vi "pathplan_vertices_send - 副本.vi"(1 "vertices":dbl[][](array[numeric])=[[5650.0, 5700.0, 5675.0, 5651.0, 5626.0, 5602.0, 5577.0, 5553.0, 5529.0, 5504.0], [1700.0, 1750.0, 1793.0, 1837.0, 1880.0, 1924.0, 1968.0, 2011.0, 2055.0, 2099.0]], 2 "distance_all":dbl, 3 "angle_all":dbl[](array[numeric])=[45.0, 119.0, 119.0, 119.0, 119.0, 119.0, 119.0, 119.0, 119.0, 0.0], 4 "speed_max":dbl, 5 "写入串口":refnum<visa-resource-name>) -> (20 "路径规划数据写入缓冲区":string)   [LabVIEW 2016]
uses:
  <vilib>/imath/engines/lvmath2/RunTimeEngine/NodeEndStatement/NIMS_NodeEndStatement_Output.vi
  <instcachedir>/0/NIMS_NodeEndStatement_Output_53EC0D466D134D7ABD903AC30B43404B.lvgen/NIMS_NodeEndStatement_Output_53EC0D466D134D7ABD903AC30B43404B_015.vi
  <instcachedir>/0/NIMS_NodeEndStatement_Output_53EC0D466D134D7ABD903AC30B43404B.lvgen/NIMS_NodeEndStatement_Output_53EC0D466D134D7ABD903AC30B43404B_011.vi
  <vilib>/imath/engines/lvmath2/RunTimeEngine/ErrorHandling/NIMS_Finalize Error.vi
  <vilib>/imath/engines/lvmath2/RunTimeEngine/IndexRead/NIMS M($,S).vi
  <instcachedir>/0/NIMS M($,S)_3E5749BBB62E49528D4765A77F1F6D98.lvgen/NIMS M($,S)_3E5749BBB62E49528D4765A77F1F6D98_000.vi
  <vilib>/imath/engines/lvmath2/RunTimeEngine/ArithmeticOperatorToken/NIMS_ArithmeticOperator_minus.vi
  <instcachedir>/0/NIMS_ArithmeticOperator_minus_E3B65B1D26A44BB184AFDC5B3F458E3D.lvgen/NIMS_ArithmeticOperator_minus_E3B65B1D26A44BB184AFDC5B3F458E3D_003.vi
  <vilib>/imath/engines/lvmath2/RunTimeEngine/ErrorHandling/NIMS_Create Error From Enums.vi
  <vilib>/imath/engines/lvmath2/RunTimeEngine/IndexRead/NIMS V(S).vi
  <instcachedir>/0/NIMS V(S)_0488751826AF41519A22953C041130DC.lvgen/NIMS V(S)_0488751826AF41519A22953C041130DC_000.vi
  <vilib>/imath/engines/lvmath2/RunTimeEngine/BuiltInFunctions/abs/NIMS_abs(signed).vi
  <instcachedir>/0/NIMS_abs(signed)_C4FCB8E6058B49B797C7C8D53CA5F6EC.lvgen/NIMS_abs(signed)_C4FCB8E6058B49B797C7C8D53CA5F6EC_000.vi
  <vilib>/imath/engines/lvmath2/RunTimeEngine/BuiltInFunctions/length/NIMS_length(GM).vi
  <instcachedir>/0/NIMS_length(GM)_47CEC356FCE0482D9BA47DC61C99F2C7.lvgen/NIMS_length(GM)_47CEC356FCE0482D9BA47DC61C99F2C7_000.vi
  <vilib>/imath/engines/lvmath2/RunTimeEngine/IndexRead/NIMS M($,R2).vi
  <instcachedir>/0/NIMS M($,R2)_D9380E19261A4ADFB2D364AF6959C6EF.lvgen/NIMS M($,R2)_D9380E19261A4ADFB2D364AF6959C6EF_001.vi
  <vilib>/imath/engines/lvmath2/RunTimeEngine/RowToken/NIMS_RowToken_M_CV.vi
  <instcachedir>/0/NIMS_RowToken_M_CV_FA79F1D1D17D44459F3ED8E09EE8B625.lvgen/NIMS_RowToken_M_CV_FA79F1D1D17D44459F3ED8E09EE8B625_000.vi
  <vilib>/imath/engines/lvmath2/RunTimeEngine/BuiltInFunctions/size/NIMS_I32=size(GM,I32).vi
  <instcachedir>/0/NIMS_I32=size(GM,I32)_122058B1B3294FAEA5DC209B92B394E4.lvgen/NIMS_I32=size(GM,I32)_122058B1B3294FAEA5DC209B92B394E4_004.vi
  <vilib>/imathl/engines/lvmath/Functions/Error Handling/Create Error.vi
  <vilib>/imath/engines/lvmath2/RunTimeEngine/RangeToken/NIMS_Range_R2 - Integer.vi
  <instcachedir>/0/NIMS_Range_R2 - Integer_89B873E74E6E489885E44F751DD9C6BF.lvgen/NIMS_Range_R2 - Integer_89B873E74E6E489885E44F751DD9C6BF_000.vi
  <vilib>/imath/engines/lvmath2/RunTimeEngine/CommandStatement/MC_CommandStatement_break.vi
  <vilib>/imath/engines/lvmath2/RunTimeEngine/BuiltInFunctions/norm/NIMS_norm(GV,DBL).vi
  <instcachedir>/0/NIMS_norm(GV,DBL)_1268AFF3C646412B8C6EA3CE75D09042.lvgen/NIMS_norm(GV,DBL)_1268AFF3C646412B8C6EA3CE75D09042_000.vi
  <instcachedir>/0/NIMS_NodeEndStatement_Output_53EC0D466D134D7ABD903AC30B43404B.lvgen/NIMS_NodeEndStatement_Output_53EC0D466D134D7ABD903AC30B43404B_010.vi
  <instcachedir>/0/NIMS_NodeEndStatement_Output_53EC0D466D134D7ABD903AC30B43404B.lvgen/NIMS_NodeEndStatement_Output_53EC0D466D134D7ABD903AC30B43404B_005.vi
  <vilib>/imath/engines/lvmath2/RunTimeEngine/BuiltInFunctions/dot/NIMS_dot(GV,GV).vi
  <instcachedir>/0/NIMS_dot(GV,GV)_B9FAA411F4494E9B94D442721014A3FA.lvgen/NIMS_dot(GV,GV)_B9FAA411F4494E9B94D442721014A3FA_000.vi
  <instcachedir>/0/NIMS_NodeEndStatement_Output_53EC0D466D134D7ABD903AC30B43404B.lvgen/NIMS_NodeEndStatement_Output_53EC0D466D134D7ABD903AC30B43404B_009.vi
panel:
  in  "y":dbl
  in  "x":dbl
  in  "angle_z":sgl
  out "angle_send":dbl[](array[numeric])
  out "vertices_send":dbl[](array[numeric])
  out "speed_send":dbl[](array[numeric])
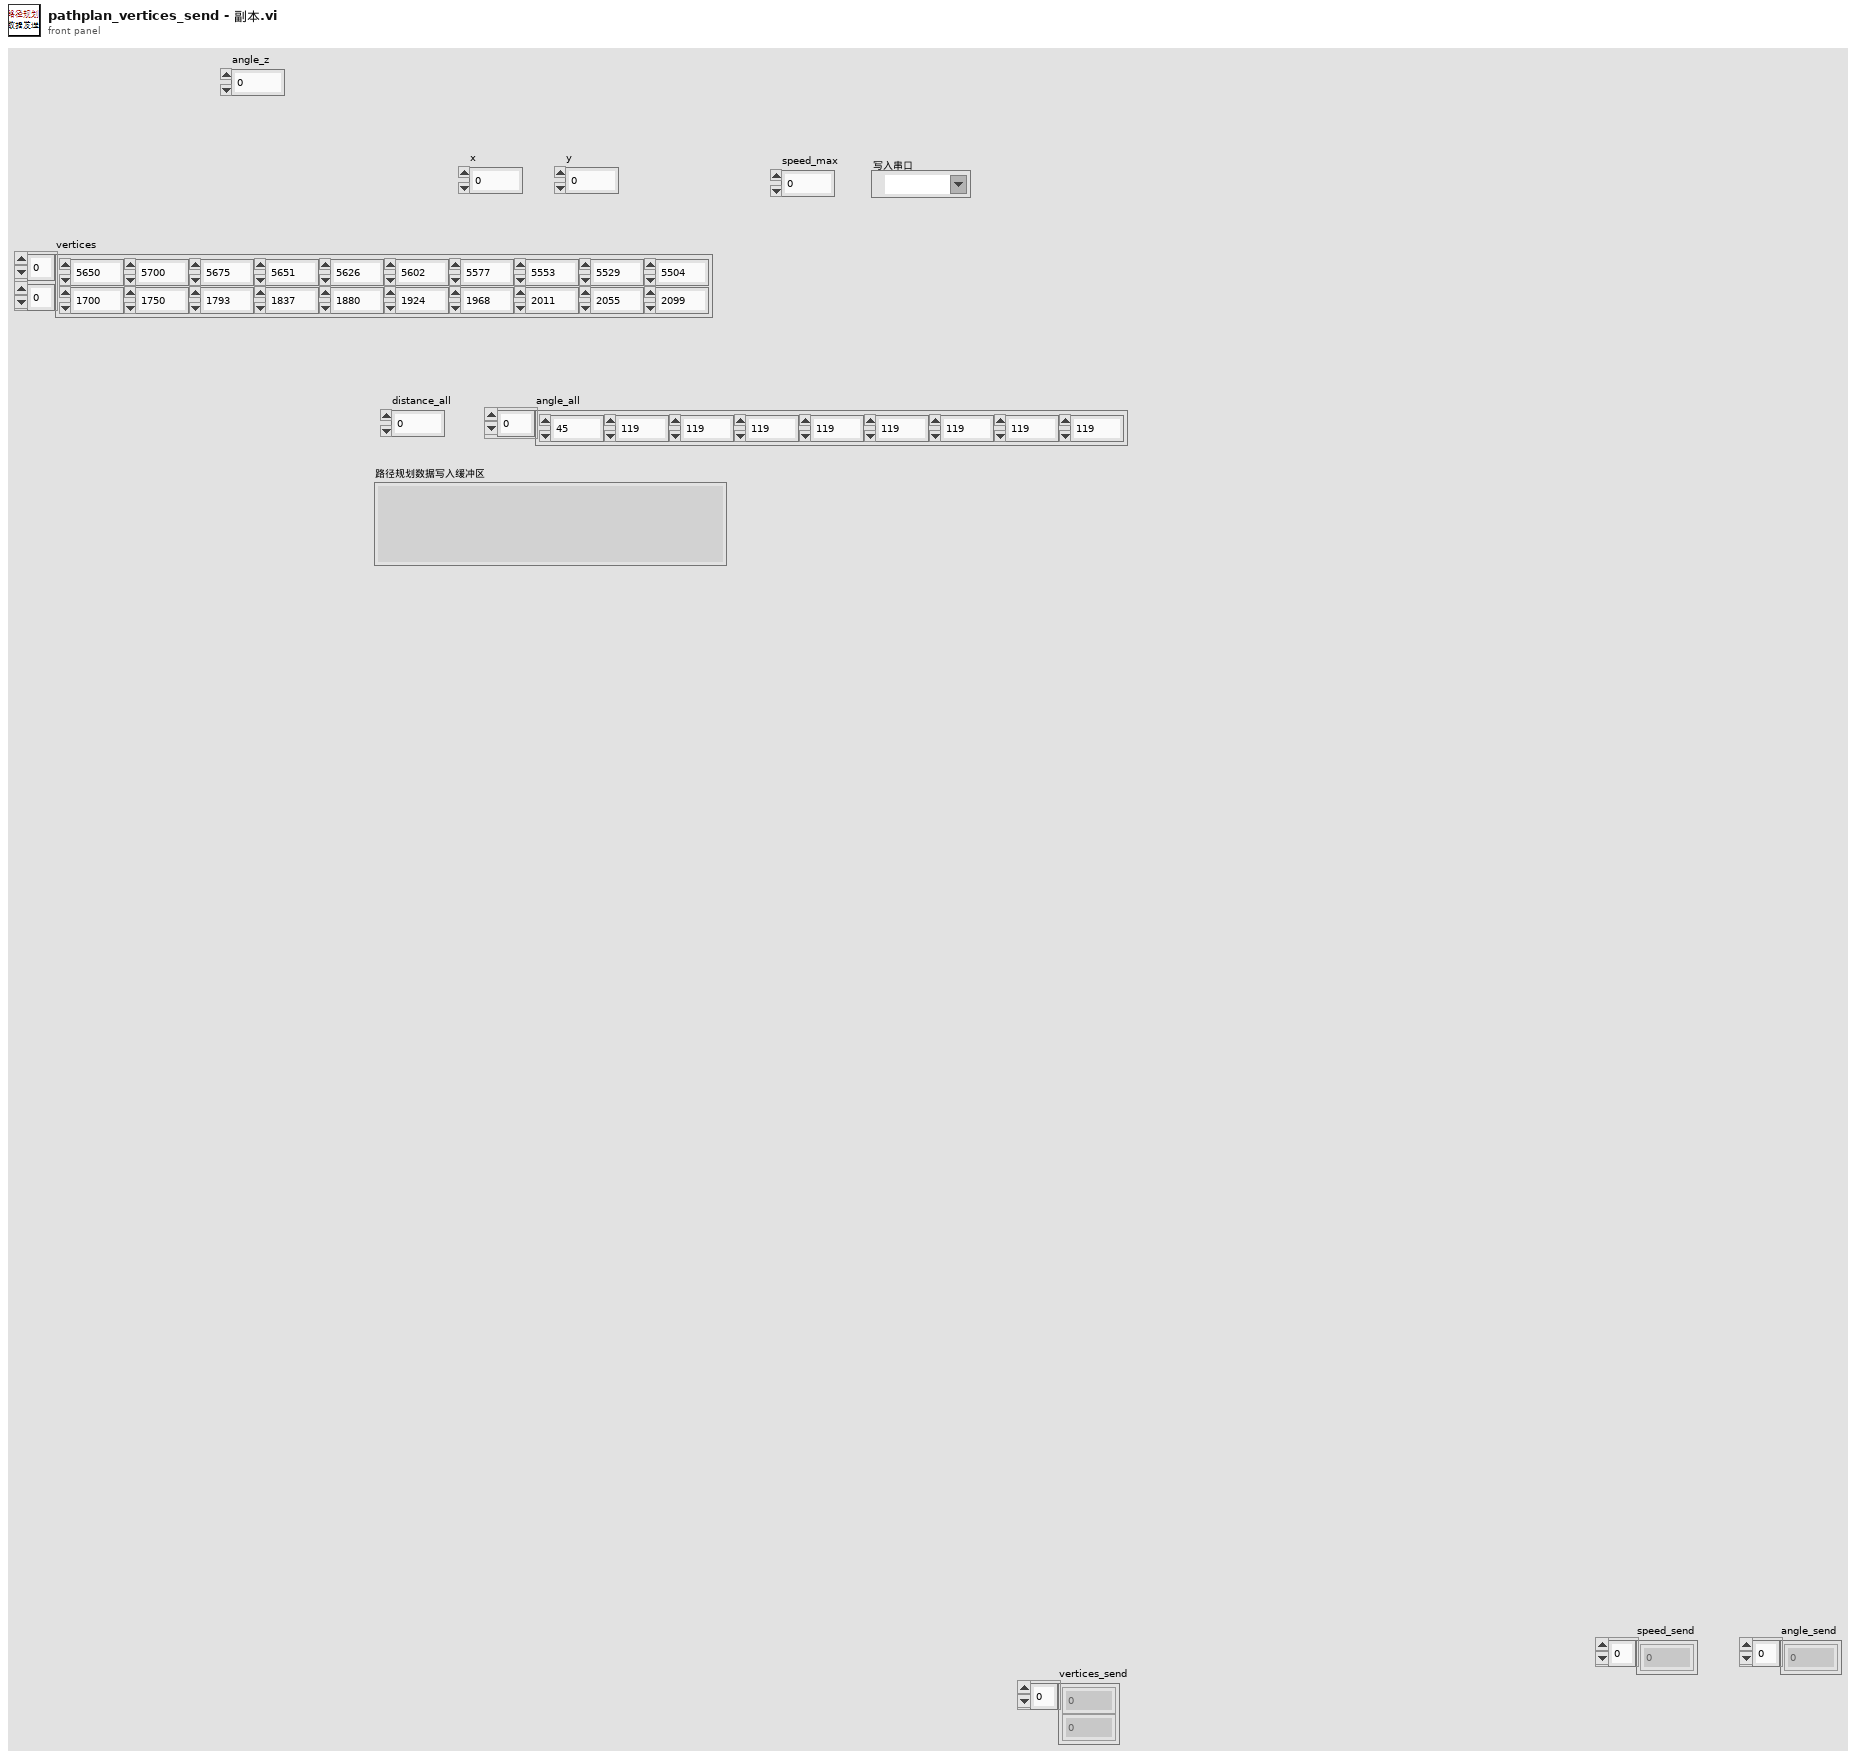
[diagram p1: front panel]
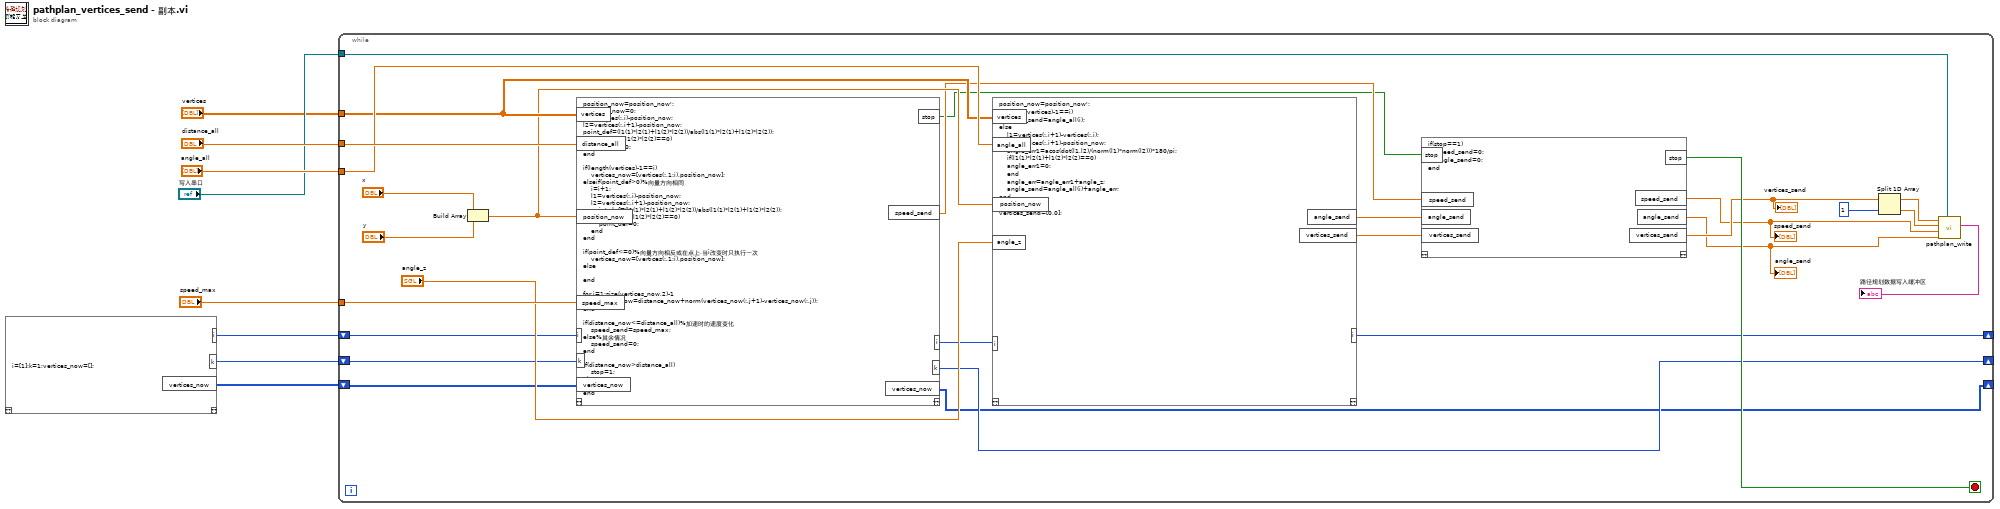
[diagram p0: block diagram]
diagram:
  n1 = mathscript code="i=[1];k=1;vertices_now=[];"() -> ("i"=w3:i32, "k"=w2:i32, "vertices_now"=w1:i32[][])  [unwired: 1 in, 1 out]
  n2 = while {
    tunnel: "vertices" -> [w34]
    tunnel: "distance_all" -> [w36]
    tunnel: "angle_all" -> [w35]
    shift-right: [w11] -> _
    shift-left: w3 -> [w13]
    tunnel: "speed_max" -> [w32]
    shift-right: [w14] -> _
    shift-left: w2 -> [w15]
    shift-right: [w9] -> _
    shift-left: w1 -> [w10]
    tunnel: "写入串口" -> [w20]
    stop <- w24 stop-if-true
    n3 = Build Array("x", "y") -> (w33:dbl[])
    n4 = mathscript code="position_now=position_now';\ndistance_now=0;\nl1=vertices(:,i)-position_now;\nl2=vertices(:,i+1)-position_now;\npoint_def=(l1(1)*l2(1)+l1(2)*l2(2))/abs(l1(1)*l2(1)+l1(2)*l2(2));\nif(l1(1)*l2(1)+l1(2)*l2(2)==0)\n    point_def=0;\nend\n\nif(length(vertices)-1==i)\n    vertices_now=[vertices(:,1:i),position_now];\nelseif(point_def>0)%向量方向相同\n    i=i+1;\n    l1=vertices(:,i)-position_now;\n    l2=vertices(:,i+1)-position_now;\n    point_def=(l1(1)*l2(1)+l1(2)*l2(2))/abs(l1(1)*l2(1)+l1(2)*l2(2));\n    if(l1(1)*l2(1)+l1(2)*l2(2)==0)\n        point_def=0;\n    end\nend\n\nif(point_def<=0)%向量方向相反或在点上,当i改变时只执行一次\n    vertices_now=[vertices(:,1:i),position_now];\nelse\n\nend\n\nfor j=1:size(vertices_now,2)-1\n    distance_now=distance_now+norm(vertices_now(:,j+1)-vertices_now(:,j));\nend\n\nif(distance_now<=distance_all)%加速时的速度变化\n    speed_send=speed_max;\nelse%其余情况\n    speed_send=0;\nend\n\nif(distance_now>distance_all)\n    stop=1;\nelse\n    stop=0;\nend"("position_now"=w33, "vertices"=w34, "distance_all"=w36, "i"=w13, "speed_max"=w32, "k"=w15, "vertices_now"=w10) -> ("k"=w14:i32, "vertices_now"=w9:i32[][], "speed_send"=w27:dbl[], "stop"=w25:bool, "i"=w12:i32)  [unwired: 1 in, 1 out]
    n5 = mathscript code="position_now=position_now';\nif(length(vertices)-1==i)\n    angle_send=angle_all(i);\nelse\n    l1=vertices(:,i+1)-vertices(:,i);\n    l2=vertices(:,i+1)-position_now;\n    angle_err1=acos(dot(l1,l2)/(norm(l1)*norm(l2)))*180/pi;\n    if(l1(1)*l2(1)+l1(2)*l2(2)==0)\n    angle_err1=0;\n    end\n    angle_err=angle_err1+angle_z;\n    angle_send=angle_all(i)+angle_err;\nend\n\nvertices_send=[0,0];"("angle_all"=w35, "vertices"=w34, "position_now"=w33, "angle_z"="angle_z", "i"=w12) -> ("i"=w11:i32, "angle_send"=w28:cdb, "vertices_send"=w26:dbl[])  [unwired: 1 in, 1 out]
    n6 = mathscript code="if(stop==1)\n    speed_send=0;\n    angle_send=0;\nend"("speed_send"=w27, "angle_send"=w28, "vertices_send"=w26, "stop"=w25) -> ("stop"=w24:bool, "angle_send"=w21:dbl[], "speed_send"=w22:dbl[], "vertices_send"=w23:dbl[])  [unwired: 1 in, 1 out]
    "speed_send" <- w22
    "vertices_send" <- w23
    "angle_send" <- w21
    n7 = Split 1D Array(array=w23, index=1 ("索引")) -> (first subarray=w30:dbl[], second subarray=w29:dbl[])
    n8 = call "pathplan_write.vi"("VISA资源名称"=w20, "angle"=w21, "v"=w22, "y"=w29, "x"=w30) -> ("路径规划数据写入缓冲区"=→"路径规划数据写入缓冲区":string)  [unwired: 6 in]
  }
